vi "Creators Created Queues.vi"(8 "Created Queue Alias":string, 9 "Priority?":bool, 10 "Msg Strategy":refnum<class "Msg Strategy.lvclass">, 11 "Base Event in":refnum<class "Base Event.lvclass">) -> (3 "Base Event out":refnum<class "Base Event.lvclass">)   [LabVIEW 2021, in "jettl.lvlib" / "Base Event.lvlib" / "Base Event.lvclass"]
uses:
  Base Event.lvclass
  C:/git/jettl/jettl/jettl/jettl/jettl.lvclass
  Msg Strategy/Msg Strategy.lvclass
  Base Event.lvclass/Base Event.ctl
  Addresses/Addresses.lvlib
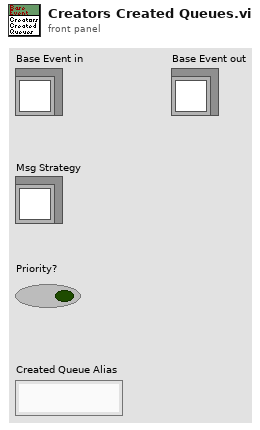
[diagram p1: front panel]
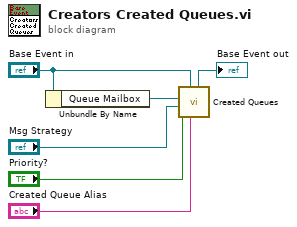
[diagram p0: block diagram]
diagram:
  n1 = Unbundle By Name("Base Event in") -> ("Queue Mailbox"=w6:refnum<data-value>)
  n2 = call "Created Queues.vi"("Created Queue Alias"="Created Queue Alias", "jettl in"="Base Event in", "Priority?"="Priority?", "Msg Strategy"="Msg Strategy", "Queue Mailbox"=w6) -> ("jettl out"=→"Base Event out":refnum<class "Base Event.lvclass">)  [unwired: 6 in]
